vi "Task 9 Prototpye Sequence Structure.vi"() -> ()   [LabVIEW 2018]
uses:
  <vilib>/Studica/Studica Toolkit/NavX/TypeDefs/Flags/Z900_navX_Flags_OpStatusTypeDef.ctl
  <vilib>/Studica/Studica Toolkit/NavX/TypeDefs/Flags/Z900_navX_Flags_CalibrationStatusTypeDef.ctl
  Underlying VI's/Modified webcam FGV/Webcam AE.ctl
  <vilib>/userdefined/High Color/IMAQdx.ctl
  Underlying VI's/I2C Master VI/Arduino_Interfacing.ctl
  Underlying VI's/I2C Master VI/I2C_MASTER_WRITE_NEW Type Def.ctl
  Underlying VI's/NavX VI/navX type def.ctl
  Underlying VI's/Motor Control VI with PID/MOTOR CONTROL WITH PID AE DATA MODE TYPE DEF.ctl
  Underlying VI's/Motor Control VI with PID/MOTOR CONTROL WITH PID AE DIRECTION TYPE DEF.ctl
  <vilib>/Studica/Studica Toolkit/Background/I2C Channel.ctl
  Underlying VI's/Elasped Timer/Elapsed timer control.ctl
  <vilib>/Studica/Studica Toolkit/NavX/NavX.lvlib
panel:
  out "NavX Readings":T1
  out "Status":T4 {"OP Status" items=["INITIALIZING", "SELFTEST_IN_PROGRESS", "ERROR", "IMU_AUTOCAL_IN_PROGRESS", "NORMAL"]; "Calibration Status" items=["IMU_CAL_STATE_MASK"=3, "IMU_CAL_STATE_INPROGRESS"=0, "IMU_CAL_STATE_ACCUMULATE"=1, "IMU_CAL_STATE_COMPLETE"=2]}
  out "Rotated to angle?":bool
  out "error out":errorcluster
  out "Colour output boolean cluster":T5
  out "Colour scan time out?":bool
  out "Acquire done?":bool
  out "Arduino Data":T6
  out "Z Stepper Position reached?":bool
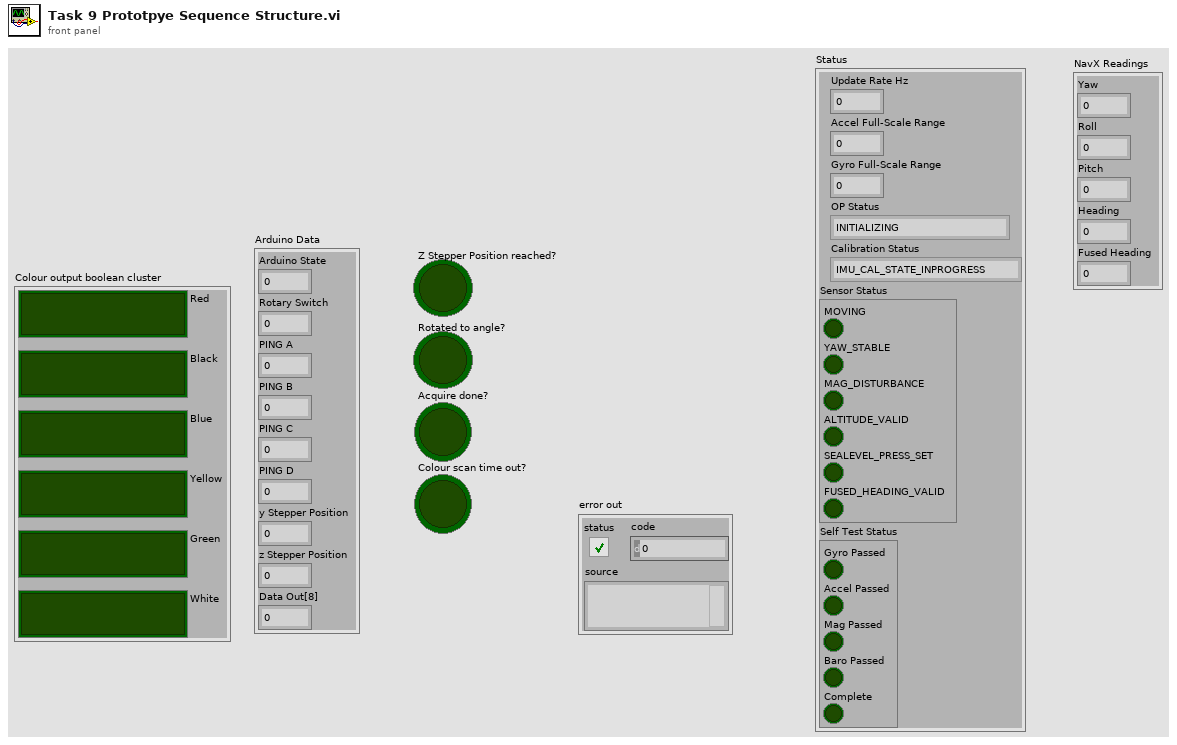
[diagram p1: front panel]
types:
  T1 = cluster{"Yaw":dbl, "Roll":dbl, "Pitch":dbl, "Heading":dbl, "Fused Heading":dbl}
  T2 = typedef "NavX.lvlib/Z900_navX_Flags_OpStatusTypeDef.ctl" = u8
  T3 = typedef "NavX.lvlib/Z900_navX_Flags_CalibrationStatusTypeDef.ctl" = u8
  T4 = cluster{"Update Rate Hz":u8, "Accel Full-Scale Range":u8, "Gyro Full-Scale Range":u16, "OP Status":T2, "Calibration Status":T3, "Sensor Status":cluster{"MOVING":bool, "YAW_STABLE":bool, "MAG_DISTURBANCE":bool, "ALTITUDE_VALID":bool, "SEALEVEL_PRESS_SET":bool, "FUSED_HEADING_VALID":bool}, "Self Test Status":cluster{"Gyro Passed":bool, "Accel Passed":bool, "Mag Passed":bool, "Baro Passed":bool, "Complete":bool}}
  T5 = cluster{"Red":bool, "Black":bool, "Blue":bool, "Yellow":bool, "Green":bool, "White":bool}
  T6 = cluster{"Arduino State":u8, "Rotary Switch":u8, "PING A":u8, "PING B":u8, "PING C":u8, "PING D":u8, "y Stepper Position":u8, "z Stepper Position":u8, "Data Out[8]":u8}
  T7 = typedef "Webcam AE.ctl" = enum16{"Initialize Camera", "Open Camera", "Continuous Acquisition", "Close Camera", "Retrieve Image", "Dispose Camera Image Buffer"}
  T8 = typedef "IMAQdx.ctl" = refnum<k21>
  T9 = typedef "I2C_MASTER_WRITE_NEW Type Def.ctl" = enum16{"Ultrasonic sensors", "Stepper origin", "zStepper 13.3k", "zStepper 13k", "zStepper 12k", "zStepper 11k", "zStepper 10k", "zStepper 9k", "zStepper 8k", "zStepper 7k", "zStepper 6k", "zStepper 5k", "zStepper 4k", "zStepper 3k", "zStepper 2k", "zStepper 1k", "zStepper 900", "zStepper 800", "zStepper 700", "zStepper 600", "zStepper 500", "zStepper 400", "zStepper 300", "zStepper 200", "zStepper 100", "zStepper 0", "yStepper control", "Open Claw", "Close Claw", "Soft Reset"}
  T10 = typedef "Arduino_Interfacing.ctl" = enum16{"Initialize", "Write to Arduino", "Read From Arduino"}
  T11 = typedef "I2C Channel.ctl" = enum16{"Not Connected", "A", "B"}
  T12 = typedef "MOTOR CONTROL WITH PID AE DIRECTION TYPE DEF.ctl" = enum16{"y-axis movement", "x-axis movement", "rotation", "stop", "reset encoders"}
  T13 = typedef "MOTOR CONTROL WITH PID AE DATA MODE TYPE DEF.ctl" = enum16{"Init AE", "Write to AE", "Read from AE"}
  T14 = typedef "navX type def.ctl" = enum16{"Get i2C reference", "Read Values", "Zero Yaw"}
  T15 = typedef "Elapsed timer control.ctl" = enum16{"Start", "Pause", "Initialize"}
  T16 = cluster{"I2C Ref Out":cluster{"I2C Channel":T11, "FPGA VI Reference Out":refnum<k20>}, "Connected":bool, "Slave Address (7-bit)":u8, "Registry":u8[]}
  T17 = cluster{"xSpeed":dbl, "ySpeed":dbl, "wSpeed":dbl, "xDistance":dbl, "yDistance":dbl, "wDistance":dbl}
  T18 = cluster{"xSpeed":bool, "ySpeed":bool, "wSpeed":bool, "xDistance":bool, "yDistance":bool, "wDistance":bool}
  T19 = typedef "IMAQ Image.ctl" = refnum<image>
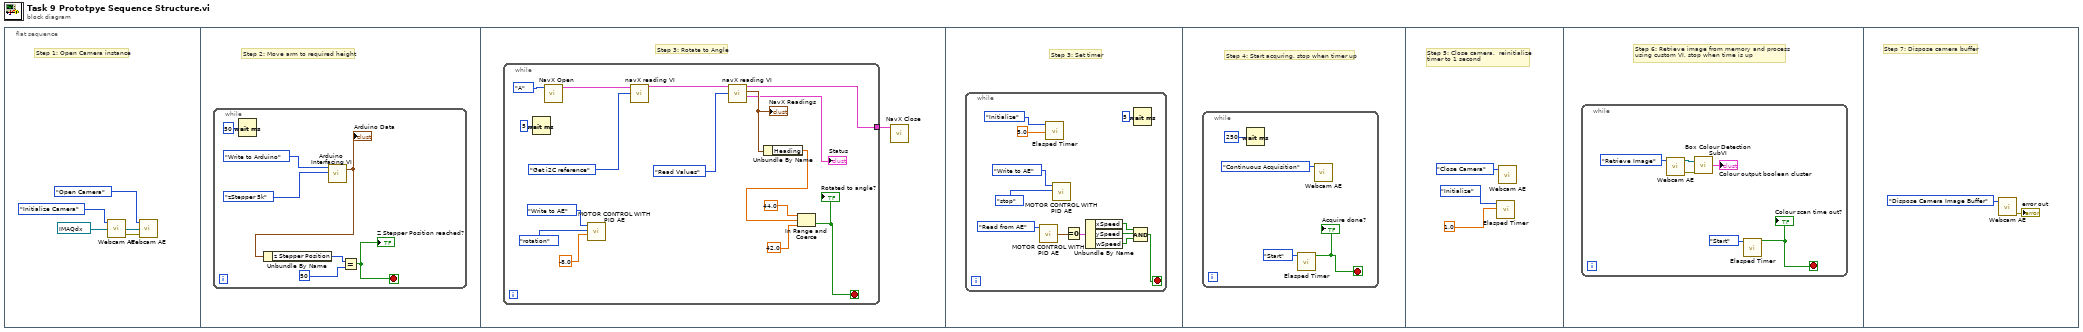
[diagram p0: block diagram]
diagram:
  n1 = flat-sequence {
    frame #0 {
      # "Step 1: Open Camera instance"
      n2 = call "Webcam AE.vi"("Session In"=T8 "cam1", "Camera states"=Webcam_AE."Initialize Camera") -> ("error out"=w4:errorcluster, "Session Out"=w5:T8)  [unwired: 1 in, 1 out]
      n3 = call "Webcam AE.vi"("error in (no error)"=w4, "Session In"=w5, "Camera states"=Webcam_AE."Open Camera") -> ()  [unwired: 3 out]
    }
    frame #1 {
      # "Step 2: Move arm to required height"
      n4 = while {
        stop <- w7 stop-if-true
        n5 = Wait (ms)(milliseconds to wait=u32 50) -> ()  [unwired: 1 out]
        n6 = call "Arduino Interfacing VI.vi"("Data to Write"=I2C_MASTER_WRITE_NEW_Type_Def."zStepper 5k", "AE Mode"=Arduino_Interfacing."Write to Arduino") -> ("Arduino Data"=w9:T6)  [unwired: 2 in, 1 out]
        "Arduino Data" <- w9
        n7 = Unbundle By Name(w9) -> ("z Stepper Position"=w6:u8)
        n8 = Equal?(x=w6, y=u8 50) -> (x = y?=w7:bool)
        "Z Stepper Position reached?" <- w7
      }
    }
    frame #2 {
      # "Step 3: Rotate to Angle"
      n9 = while {
        tunnel: [w26] -> w13
        stop <- w17 stop-if-true
        n10 = Wait (ms)(milliseconds to wait=u32 5 ("millisecond timer value")) -> ()  [unwired: 1 out]
        n11 = call <vilib>:"NavX Open.vi"("I2C Channel"=I2C_Channel."A") -> ("NavX Info"=w14:T16)  [unwired: 9 in, 1 out]
        n12 = call "MOTOR CONTROL WITH PID AE.vi"("Speed"=-8.0, "Direction"=MOTOR_CONTROL_WITH_PID_AE_DIRECTION_TYPE_DEF."rotation", "AE Mode"=MOTOR_CONTROL_WITH_PID_AE_DATA_MODE_TYPE_DEF."Write to AE") -> ()  [unwired: 1 in, 1 out]
        n13 = call "navX reading VI.vi"("NavX Info In"=w14, "Mode"=navX_type_def."Get i2C reference") -> ("NavX Info Out"=w29:T16)  [unwired: 1 in, 3 out]
        n14 = call "navX reading VI.vi"("NavX Info In"=w29, "Mode"=navX_type_def."Read Values") -> ("NavX Info Out"=w26:T16, "NavX Readings"=w25:T1, "Status"=→"Status":T4)  [unwired: 1 in, 1 out]
        "NavX Readings" <- w25
        n15 = Unbundle By Name(w25) -> ("Heading"=w18:dbl)
        n16 = In Range and Coerce(upper limit=44.0, x=w18, lower limit=42.0) -> (In Range?=w17:bool)  [unwired: 1 out]
        "Rotated to angle?" <- w17
      }
      n17 = call <vilib>:"NavX Close.vi"("NavX Info In"=w13) -> ()  [unwired: 10 in, 1 out]
    }
    frame #3 {
      # "Step 3: Set timer"
      n18 = while {
        stop <- w31 stop-if-true
        n19 = call "MOTOR CONTROL WITH PID AE.vi"("AE Mode"=MOTOR_CONTROL_WITH_PID_AE_DATA_MODE_TYPE_DEF."Read from AE") -> ("Speed & distance"=w36:T17)  [unwired: 3 in]
        n20 = call "Elasped Timer.vi"("Time Setting"=5.0, "Action"=Elapsed_timer_control."Initialize") -> ()  [unwired: 6 in, 4 out]
        n21 = call "MOTOR CONTROL WITH PID AE.vi"("Direction"=MOTOR_CONTROL_WITH_PID_AE_DIRECTION_TYPE_DEF."stop", "AE Mode"=MOTOR_CONTROL_WITH_PID_AE_DATA_MODE_TYPE_DEF."Write to AE") -> ()  [unwired: 2 in, 1 out]
        n22 = Equal To 0?(x=w36) -> (x = 0?=w35:T18)
        n23 = Unbundle By Name(w35) -> ("xSpeed"=w34:bool, "ySpeed"=w33:bool, "wSpeed"=w32:bool)
        n24 = Wait (ms)(milliseconds to wait=u32 5 ("millisecond timer value")) -> ()  [unwired: 1 out]
        n25 = Compound Arithmetic op=AND(w34, w33, w32) -> (w31:bool)
      }
    }
    frame #4 {
      # "Step 4: Start acquring, stop when timer up"
      n26 = while {
        stop <- w42 stop-if-true
        n27 = Wait (ms)(milliseconds to wait=u32 250 ("millisecond timer value")) -> ()  [unwired: 1 out]
        n28 = call "Elasped Timer.vi"("Action"=Elapsed_timer_control."Start") -> ("Time Out?!"=w42:bool)  [unwired: 7 in, 3 out]
        "Acquire done?" <- w42
        n29 = call "Webcam AE.vi"("Camera states"=Webcam_AE."Continuous Acquisition") -> ()  [unwired: 2 in, 3 out]
      }
    }
    frame #5 {
      # "Step 5: Close camera,  reinitialize \ntimer to 1 second"
      n30 = call "Elasped Timer.vi"("Time Setting"=1.0, "Action"=Elapsed_timer_control."Initialize") -> ()  [unwired: 6 in, 4 out]
      n31 = call "Webcam AE.vi"("Camera states"=Webcam_AE."Close Camera") -> ()  [unwired: 2 in, 3 out]
    }
    frame #6 {
      # "Step 6: Retrieve image from memory and process\nusing custom VI, stop when time is up"
      n32 = while {
        stop <- w49 stop-if-true
        n33 = call "Webcam AE.vi"("Camera states"=Webcam_AE."Retrieve Image") -> ("error out"=w51:errorcluster, "Image Out"=w52:T19)  [unwired: 2 in, 1 out]
        n34 = call "Box Colour Detection SubVI.vi"("Image In"=w52, "Error In"=w51) -> ("Colour output boolean cluster"=→"Colour output boolean cluster":T5)  [unwired: 2 out]
        n35 = call "Elasped Timer.vi"("Action"=Elapsed_timer_control."Start") -> ("Time Out?!"=w49:bool)  [unwired: 7 in, 3 out]
        "Colour scan time out?" <- w49
      }
    }
    frame #7 {
      # "Step 7: Dispose camera buffer"
      n36 = call "Webcam AE.vi"("Camera states"=Webcam_AE."Dispose Camera Image Buffer") -> ("error out"=→"error out":errorcluster)  [unwired: 2 in, 2 out]
    }
  }
